vi "Write Cntrller Reference.vi"(8 "error in (no error)":errorcluster, 10 "Cntrller Reference":refnum<k24>, 11 "Newport in":refnum<class "Newport.lvclass">) -> (0 "error out":errorcluster, 3 "Newport out":refnum<class "Newport.lvclass">)   [LabVIEW 2018, in "Newport.lvlib" / "Newport.lvclass"]
uses:
  Newport.lvclass
  Newport.XPS.CommandInterface
  Newport.lvclass/Newport.ctl
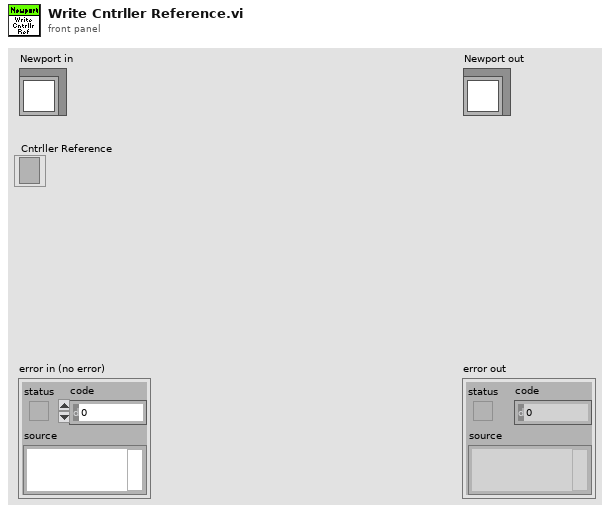
[diagram p1: front panel]
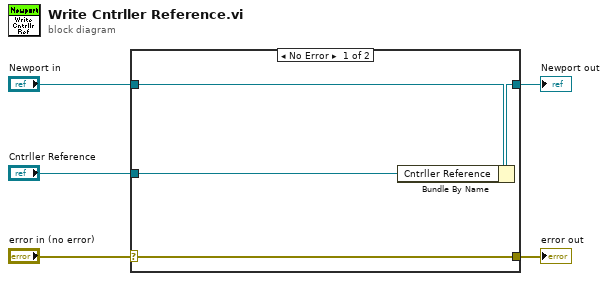
[diagram p0: block diagram]
diagram:
  n1 = case shown="No Error" "error in (no error)" {
    selector: "error in (no error)" -> [w9 w10]
    tunnel: [w9 w10] -> w4
    tunnel: [w7 w11] -> w2
    tunnel: "Newport in" -> [w8 w11]
    tunnel: "Cntrller Reference" -> [w6 _]
    frame No Error {
      n2 = Bundle By Name(cluster=w8, "Cntrller Reference"=w6) -> (w7:refnum<class "Newport.lvclass">)
    }
    frame Error {
    }
  }
  "error out" <- w4
  "Newport out" <- w2
